vi "ADC_SetConfig.vi"(8 "error in (no error)":errorcluster, 9 "ConfigBufSize":u32 format="%.0x", 10 "pConfigBuf":u8[](array[numeric]), 11 "DeviceIndex":u32) -> (0 "error out":errorcluster, 2 "ConfigBufSize":u32)   [LabVIEW 8.6]
doc: "unsigned long ADC_SetConfig(\nunsigned long DeviceIndex - number from 0-31 indicating to which device you wish to set the\nA/D configuration\nunsigned char *pConfigBuf - a pointer to the first of an array of configuration bytes\nunsigned long *ConfigBufSize - a pointer to a variable holding the number of configuration bytes\nto write. Will be set to the number of configuration bytes written\n)\nConfiguration bytes for analog input boards(the USB-AI16-16 family) are as follows:\n[00] … [0F] [10] [11] [12] [13]\nChannel 0\nGain Code … Channel 15\nGain Code\nCalibration\nCode\nTrigger &\nCounter Clock\nStart & End\nChannel Oversample\nA configuration of all zeroes is close to an \"ordinary\" use; you'll likely want to set external or\ntimer trigger, and start and end channels.\nGain codes (config bytes 00-0F) for analog input boards(the USB-AI16-16 family) are as\nfollows:\nGain Code 00 01 02 03 04 05 06 07\nRange 0-10V ±10V 0-5V ±5V 0-2V ±2V 0-1V ±1V\nFor ADC_SetConfig (only), add 08 to the gain code for channel 0-7 to pair it with the respective\nchannel 8-15 in differential mode.\nCalibration codes (config byte 10) for analog input boards(the USB-AI16-16 family) are as\nfollows:\nCal. Code 00 01 03\nEffect Acquire\nNormal Data\nAcquire Cal. Ground\n(0.0114V @ 0-10V)\nAcquire Cal. Reference\n(9.9V @ 0-10V)\nTrigger & counter clock bits (config byte 11) for analog input boards(the USB-AI16-16 family)\nare as follows:\nBit 7 6 5 4 3 2 1 0\nValue Reserved, use 0 CTR0\nEXT\nFalling\nEdge Scan External\nTrigger\nTimer\nTrigger\n• If CTR0 EXT is set, counter 0 is externally-triggered; otherwise, counter 0 is triggered by the\nonboard 10MHz clock.\n• If Falling Edge is set, A/D is triggered by the falling edge of its trigger source; otherwise, A/D\nis triggered by the rising edge of its trigger source.\n• If Scan is set, a single A/D trigger will acquire all channels from start to end, oversampling if so\nconfigured, at maximum speed. Otherwise, a single A/D trigger will cause a single acquisition,\n\"walking\" through oversamples and channels.\n22\n• If External Trigger is set, the external A/D trigger pin is an A/D trigger source. Otherwise, it's\nignored. (Immediate (software) triggering is always an A/D trigger source, as well.)\n• If Timer Trigger is set, counter 2 is an A/D trigger source. Otherwise, it's ignored.\nStart & end channel (config byte 12) for analog input boards(the USB-AI16-16 family) are the\nstart channel (0-F) in bits 0-3, and the end channel (0-F) in bits 4-7. If the end channel is less\nthan the start channel, then the board's behavior is unspecified.\nOversample (config byte 13) for analog input boards(the USB-AI16-16 family) is a number\nindicating how many extra samples should be acquired from each channel before moving on to\nthe next. In a noisy environment, the samples can be averaged together by software to effectively\nreduce noise."
uses:
  Windows/System32/AIOUSB.dll
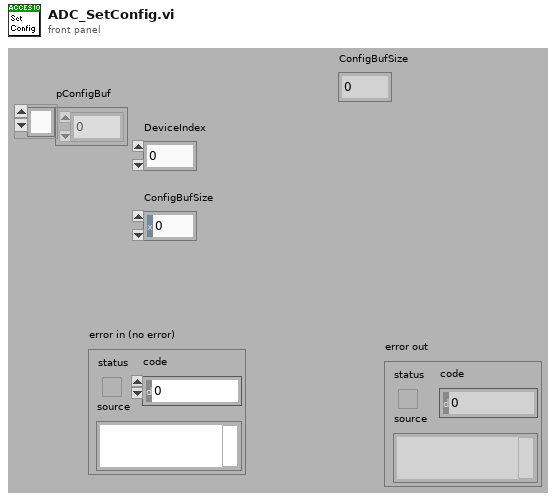
[diagram p1: front panel]
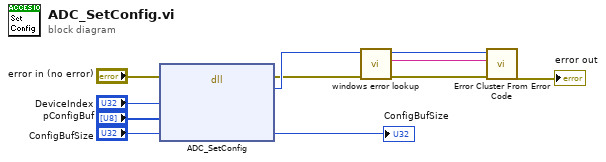
[diagram p0: block diagram]
diagram:
  n1 = dll-call lib="C:/Windows/System32/AIOUSB.dll" fn="ADC_SetConfig"(error in="error in (no error)", "DeviceIndex"="DeviceIndex", "pConfigBuf"="pConfigBuf", "ConfigBufSize"="ConfigBufSize") -> (error out=w2:errorcluster, "return type"=w3:u32, "ConfigBufSize"=→"ConfigBufSize":u32)  [unwired: 4 in, 1 out]
  n2 = call "windows error lookup.vi"("error in (no error)"=w2, "Error Code"=w3) -> ("error out"=w1:errorcluster, "error message (\"\")"=w4:string)  [unwired: 8 in]
  n3 = call <vilib>:"Error Cluster From Error Code.vi"("error in (no error)"=w1, "error message (\"\")"=w4, "error code (0)"=w3) -> ("error out"=→"error out":errorcluster)  [unwired: 6 in]
